vi "Equal Value Comparison.vi"(8 "error in (no error)":errorcluster, 9 "Y":variant, 10 "X":variant) -> (0 "error out":errorcluster, 2 "Equal Values?":bool)   [LabVIEW 2009, in "Caraya.lvlib" / "Assert.lvclass"]
uses:
  classes/Assert/Assert.lvclass
  <vilib>/Utility/VariantDataType/Type.ctl
  <vilib>/Utility/VariantDataType/VariantType.lvlib
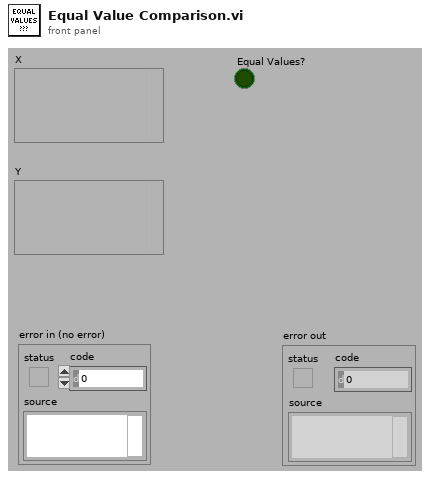
[diagram p1: front panel]
types:
  T1 = typedef "VariantType.lvlib/Type.ctl" = enum8{"Invalid Type", "Void", "I8", "I16", "I32", "I64", "U8", "U16", "U32", "U64", "Single Float", "Double Float", "Extended Float", "Single Complex", "Double Complex", "Extended Complex", "Enum U8", "Enum U16", "Enum U32", "Enum U64", "Single Float With Unit", "Double Float With Unit", "Extended Float With Unit", "Single Complex with Unit", "Double Complex with Unit", "Extended Complex with Unit", "Boolean", "String", "Path", "Picture", "Tag", "Array", "Cluster", "Variant", "LV Variant", "Waveform", "Timestamp", "Digital Waveform", "Digital Data", "ExpressData", "Refnum", "External Data", "VI", "Poly VI", "LabVIEW Class Instance", "Fixed Point"}
  T2 = typedef "Physical Units__ogtk.ctl" = cluster{"Base Units":enum16{"radian", "steradian", "second", "meter", "kilogram", "ampere", "kelvin", "mole", "candela"}, "Exponent":i16}
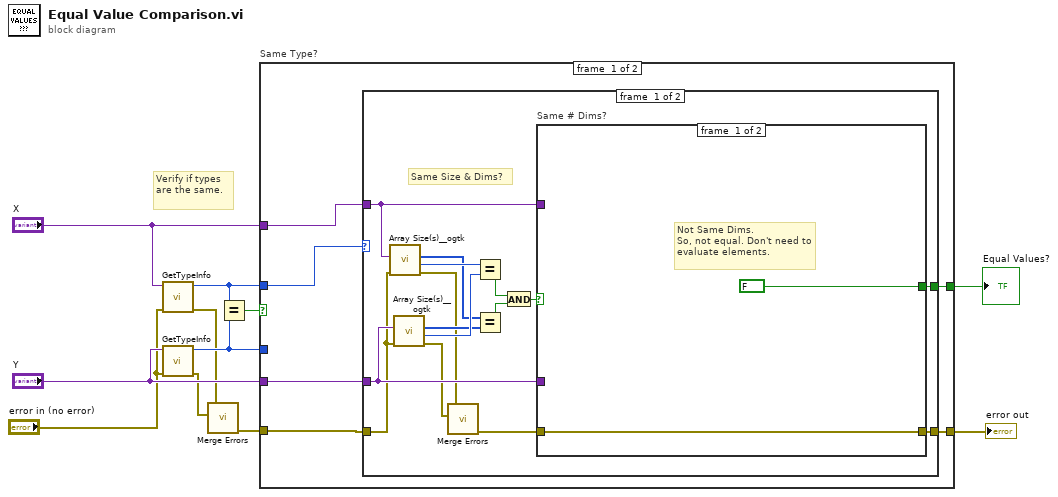
[diagram p0: block diagram]
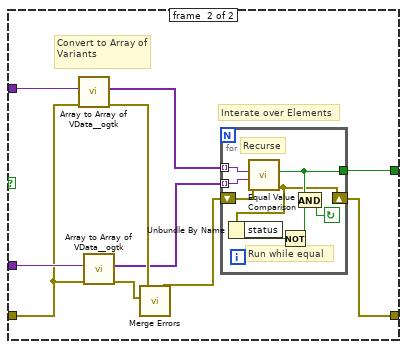
[diagram p2: hidden frame]
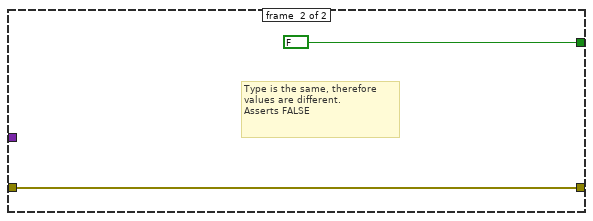
[diagram p3: hidden frame]
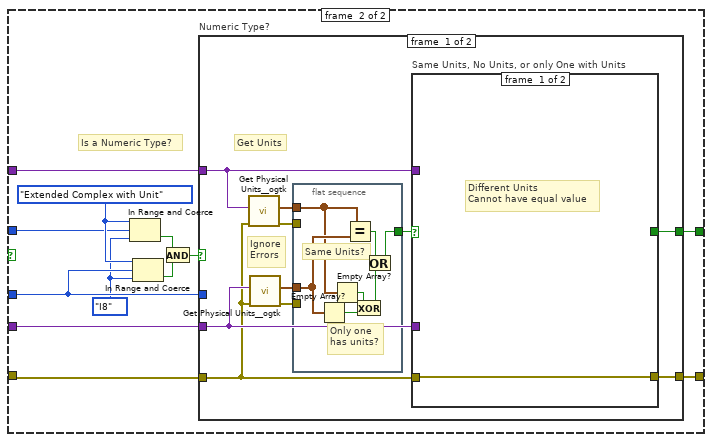
[diagram p4: hidden frame]
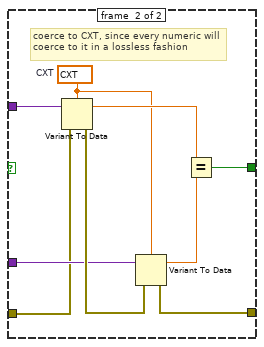
[diagram p5: hidden frame]
diagram:
  # "Verify if types are the same."
  n1 = call <vilib>:"GetTypeInfo.vi"("error in (no error)"="error in (no error)", "Variant"="X") -> ("error out"=w3:errorcluster, "Type Enum"=w5:T1)  [unwired: 5 in, 3 out]
  n2 = call <vilib>:"GetTypeInfo.vi"("error in (no error)"="error in (no error)", "Variant"="Y") -> ("error out"=w2:errorcluster, "Type Enum"=w4:T1)  [unwired: 5 in, 3 out]
  n3 = call <vilib>:"Merge Errors.vi"("error in 2 (no error)"=w2, "error in 1 (no error)"=w3) -> ("error out"=w1:errorcluster)  [unwired: 5 in]
  n4 = Equal?(x=w5, y=w4) -> (x = y?=w6:bool)
  n5 = case "Same Type?" shown="False" w6 {
    tunnel: "X" -> [w15 w66]
    tunnel: "Y" -> [w14 w65]
    tunnel: [w17 w64] -> w10
    tunnel: w5 -> [w16 w56]
    tunnel: w4 -> [_ w61]
    tunnel: w1 -> [w13 w63]
    tunnel: [w12 w62] -> w7
    frame #0 {
      n6 = case shown="\"Array\"" w16 {
        tunnel: [w32 FALSE] -> w17
        tunnel: w15 -> [w28 _]
        tunnel: w14 -> [w29 _]
        tunnel: w13 -> [w27 w53]
        tunnel: [w31 w53] -> w12
        frame #0 {
          # "Same Size & Dims?"
          n7 = call <userlib>:"Array Size(s)__ogtk.vi"("error in (no error)"=w27, "Array"=w28) -> ("error out"=w21:errorcluster, "N dims"=w25:u32, "Size(s)"=w23:u32[])  [unwired: 7 in]
          n8 = call <userlib>:"Array Size(s)__ogtk.vi"("error in (no error)"=w27, "Array"=w29) -> ("error out"=w26:errorcluster, "N dims"=w24:u32, "Size(s)"=w22:u32[])  [unwired: 7 in]
          n9 = call <vilib>:"Merge Errors.vi"("error in 2 (no error)"=w26, "error in 1 (no error)"=w21) -> ("error out"=w30:errorcluster)  [unwired: 5 in]
          n10 = Equal?(x=w25, y=w24) -> (x = y?=w19:bool)
          n11 = Equal?(x=w23, y=w22) -> (x = y?=w20:bool)
          n12 = And(x=w19, y=w20) -> (x .and. y?=w18:bool)
          n13 = case "Same # Dims?" shown="True" w18 {
            tunnel: [FALSE ("Equal Values?") w44] -> w32
            tunnel: w28 -> [_ w43]
            tunnel: w29 -> [_ w42]
            tunnel: [w33 w41] -> w31
            tunnel: w30 -> [w33 w40]
            frame #0 {
              # "Not Same Dims.\nSo, not equal. Don't need to evaluate elements."
            }
            frame #1 {
              # "Interate over Elements"
              # "Convert to Array of Variants"
              n14 = call <userlib>:"Array to Array of VData__ogtk.vi"("error in (no error)"=w40, "MultiD Array"=w43) -> ("error out"=w37:errorcluster, "1D Array of Variants"=w38:variant[])  [unwired: 8 in]
              n15 = call <userlib>:"Array to Array of VData__ogtk.vi"("error in (no error)"=w40, "MultiD Array"=w42) -> ("error out"=w36:errorcluster, "1D Array of Variants"=w35:variant[])  [unwired: 8 in]
              n16 = call <vilib>:"Merge Errors.vi"("error in 2 (no error)"=w36, "error in 1 (no error)"=w37) -> ("error out"=w39:errorcluster)  [unwired: 5 in]
              n17 = for {
                tunnel: w38 -> [w52] mode=indexing
                tunnel: w35 -> [w51] mode=indexing
                tunnel: [w47] -> w44
                shift-right: [w45] -> w41
                shift-left: w39 -> [w50]
                stop <- w46 continue-if-true
                # "Run while equal"
                # "Recurse"
                n18 = call "Equal Value Comparison.vi"("error in (no error)"=w50, "Y"=w51, "X"=w52) -> ("error out"=w45:errorcluster, "Equal Values?"=w47:bool)  [unwired: 7 in]
                n19 = Unbundle By Name(w45) -> ("status"=w48:bool)
                n20 = Not(x=w48) -> (.not. x?=w49:bool)
                n21 = And(x=w47, y=w49) -> (x .and. y?=w46:bool)
              }
            }
          }
        }
        frame #1 {
          # "Type is the same, therefore values are different.\nAsserts FALSE"
        }
      }
    }
    frame #1 {
      w59 = Type."I8" ("Type Enum")
      w60 = Type."Extended Complex with Unit" ("Type Enum")
      # "Is a Numeric Type?"
      n22 = In Range and Coerce(upper limit=w60, x=w56, lower limit=w59) -> (In Range?=w58:bool)  [unwired: 1 out]
      n23 = In Range and Coerce(upper limit=w60, x=w61, lower limit=w59) -> (In Range?=w57:bool)  [unwired: 1 out]
      n24 = And(x=w58, y=w57) -> (x .and. y?=w55:bool)
      n25 = case "Numeric Type?" shown="True" w55 {
        tunnel: w66 -> [w74 _]
        tunnel: w65 -> [w73 _]
        tunnel: w61 -> [_ _]
        tunnel: [w76 _] -> w64
        tunnel: w63 -> [w72 w94]
        tunnel: [w75 w94] -> w62
        frame #0 {
          # "Get Units"
          # "Ignore\nErrors"
          n26 = call <userlib>:"Get Physical Units__ogtk.vi"("error in (no error)"=w72, "Float or Array of Floats"=w74) -> ("error out"=w71:errorcluster, "Physical Units"=w69:T2[])  [unwired: 8 in]
          n27 = call <userlib>:"Get Physical Units__ogtk.vi"("error in (no error)"=w72, "Float or Array of Floats"=w73) -> ("error out"=w70:errorcluster, "Physical Units"=w68:T2[])  [unwired: 8 in]
          n28 = flat-sequence {
            tunnel: w71 -> [_]
            tunnel: w70 -> [_]
            tunnel: w69 -> [w92]
            tunnel: w68 -> [w93]
            tunnel: [w87] -> w67
            frame #0 {
              # "Same Units?"
              # "Only one\nhas units?"
              n29 = Empty Array?(array=w93) -> (empty?=w91:bool)
              n30 = Empty Array?(array=w92) -> (empty?=w90:bool)
              n31 = Equal?(x=w92, y=w93) -> (x = y?=w88:bool)
              n32 = Exclusive Or(1:w91, 2:w90) -> (0:w89:bool)
              n33 = Or(x=w88, y=w89) -> (x .or. y?=w87:bool)
            }
          }
          n34 = case "Same Units, No Units, or only One with Units" shown="True" w67 {
            tunnel: [_ w86] -> w76
            tunnel: [w77 w85] -> w75
            tunnel: w74 -> [_ w80]
            tunnel: w73 -> [_ w79]
            tunnel: w72 -> [w77 w78]
            frame #0 {
              # "Different Units\nCannot have equal value"
            }
            frame #1 {
              w81 = cxt 0.0+0.0i  # CXT
              # "coerce to CXT, since every numeric will coerce to it in a lossless fashion"
              n35 = Variant To Data(error in=w78, Variant=w80, type=w81) -> (error out=w82:errorcluster, data=w84:cxt)
              n36 = Variant To Data(error in=w82, Variant=w79, type=w81) -> (error out=w85:errorcluster, data=w83:cxt)
              n37 = Equal?(x=w84, y=w83) -> (x = y?=w86:bool)
            }
          }
        }
        frame #1 {
          # "All non-integer representations must be of same type to potentially assert True"
        }
      }
    }
  }
  "Equal Values?" <- w10
  "error out" <- w7
